vi "7_SystemCalls.vi"() -> ()   [LabVIEW 2012]
panel:
  out "BotSpeak":string="SYSTEM freq,12,4\nSET var,3\nSYSTEM var,2,5\nGET freq\nSCRIPT\nSET DIO[13],0\nSYSTEM var2,13,2\nWAITµs 1.000000\nSET DIO[13],1\nend\nENDSCRIPT\nRUN&WAIT 0\nSCRIPT\nSET DIO[13],0\nSYSTEM freq,10,4\nSET answer,freq\nSUB answer,2\nend\nENDSCRIPT\nRUN&WAIT 0\nGET var2\nGET freq\nGET answer\n\n"
  out "expected response":string="3\r\n2\r\n12\r\nstart script\r\n \r\n \r\n \r\n \r\n \r\nend script\r\n.....\nDone\r\nstart script\r\nend script\r\n.....\nDone\r\n13\r\n10\r\n8\r\n"
  out "response":string="3\r\n2\r\n12\r\nstart script\r\n \r\n \r\n \r\n \r\n \r\nend script\r\n.....\nDone\r\nstart script\r\nend script\r\n.....\nDone\r\n13\r\n10\r\n8\r\n"
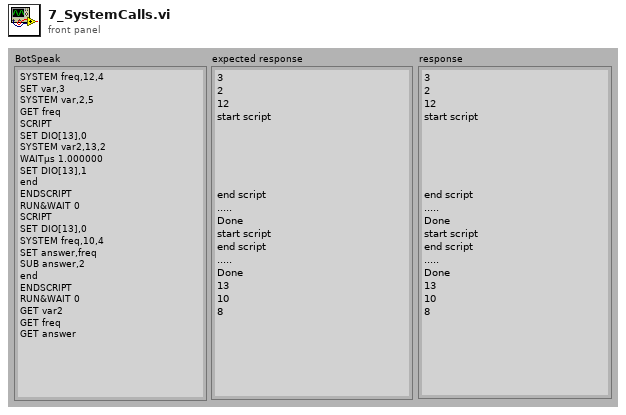
[diagram p1: front panel]
types:
  T1 = typedef "BotSpeak_Control.ctl" = cluster{"Address":string, "Reply EOF":string, "Hardware":path, "Retries":i8, "Timeout":i32}
  T2 = typedef "URAPI_Control.ctl" = cluster{"Script":string, "Whiles":u8[], "Ifs":u8[], "Supress Err":bool, "Errors":string}
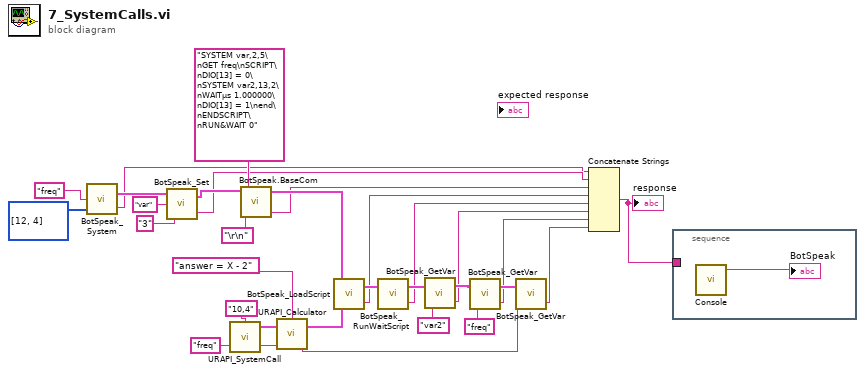
[diagram p0: block diagram]
diagram:
  n1 = call <userlib>:"BotSpeak_System.vi"("Values sent"=i16[] [12, 4], "Variable In"="freq") -> ("response"=w1:string, "Bot Settings"=w9:T1)  [unwired: 1 in]
  n2 = call <userlib>:"BotSpeak_Set.vi"("value"="3", "Variable In"="var", "Bot Settings"=w9) -> ("response"=w16:string, "Bot Settings"=w28:T1)
  n3 = call <userlib>:"URAPI_SystemCall.vi"("Variable for reply"="freq", "System call in"="10,4") -> ("Variable Out"=w3:string, "URAPI Script"=w6:T2)  [unwired: 2 in]
  n4 = call <userlib>:"BotSpeak.BaseCom.vi"("Termination"="\r\n", "command"="SYSTEM var,2,5\nGET freq\nSCRIPT\nDIO[13] = 0\nSYSTEM var2,13,2\nWAITµs 1.000000\nDIO[13] = 1\nend\nENDSCRIPT\nRUN&WAIT 0" ("String"), "Bot Settings in"=w28) -> ("response"=w15:string, "Bot Settings out"=w24:T1)  [unwired: 2 in]
  n5 = call <userlib>:"URAPI_Calculator.vi"("X"=w3, "URAPI Script"=w6, "Formula"="answer = X - 2") -> ("Variable Out"=w17:string, "URAPI Script"=w25:T2)  [unwired: 1 in]
  n6 = call <userlib>:"BotSpeak_LoadScript.vi"("URAPI Script"=w25, "Bot Settings"=w24) -> ("total response"=w14:string, "Bot Settings"=w23:T1)
  n7 = call <userlib>:"BotSpeak_RunWaitScript.vi"("Bot Settings"=w23) -> ("response"=w13:string, "Bot Settings"=w22:T1)  [unwired: 1 in]
  n8 = call <userlib>:"BotSpeak_GetVar.vi"("Variable In"="var2", "Bot Settings"=w22) -> ("value"=w12:string, "Bot Settings out"=w19:T1)
  n9 = call <userlib>:"BotSpeak_GetVar.vi"("Variable In"="freq", "Bot Settings"=w19) -> ("value"=w11:string, "Bot Settings out"=w18:T1)
  n10 = call <userlib>:"BotSpeak_GetVar.vi"("Variable In"=w17, "Bot Settings"=w18) -> ("value"=w10:string)  [unwired: 1 out]
  n11 = Concatenate Strings(w1, w16, w15, w14, w13, w12, w11, w10) -> (w2:string)
  "response" <- w2
  n12 = stacked-sequence {
    tunnel: w2 -> [_]
    frame #0 {
      n13 = call <userlib>:"Console.vi"() -> ("BotSpeak"=→"BotSpeak":string)  [unwired: 4 in, 1 out]
    }
  }
